vi "Configure Trigger (CAN).vi"(0 "VISA resource name":refnum<visa-resource-name>, 1 "Identifier":T2={"ID Mode (0: Standard)"=0, "ID Value (XXXXXXXXXXX)"="XXXXXXXXXXX"} {"ID Mode (0: Standard)" items=["Standard", "Extended"]}, 2 "Data":T1={"Data Size (1)"=1, "Data Value (XXXXXXXX)"="XXXXXXXX"}, 5 "Trigger Source (9: Bus 1)":u16(ring)=9 items=["Bus 1"=9, "Bus 2"=10, "Bus 3"=11, "Bus 4"=12], 7 "Condition (0: Start of Frame)":u16(ring) items=["Start of Frame", "Type of Frame", "Identifier", "Data", "ID & Data", "End of Frame", "Missing Ack"], 9 "Frame Type (0: Data)":u16(ring) items=["Data", "Remote", "Error", "Overload"], 11 "error in (no error)":errorcluster) -> (4 "VISA resource name out":refnum<visa-resource-name>, 15 "error out":errorcluster)   [LabVIEW 2013, in "Tektronix DPO MSO 2000 4000 Series.lvlib"]
doc: "Configures CAN trigger settings for an oscilloscope."
uses:
  Tektronix DPO MSO 2000 4000 Series.lvlib
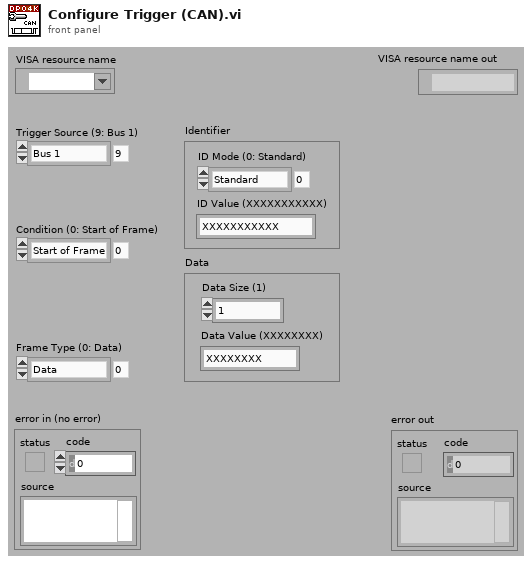
[diagram p1: front panel]
types:
  T1 = cluster{"Data Size (1)":i32, "Data Value (XXXXXXXX)":string}
  T2 = cluster{"ID Mode (0: Standard)":u16, "ID Value (XXXXXXXXXXX)":string}
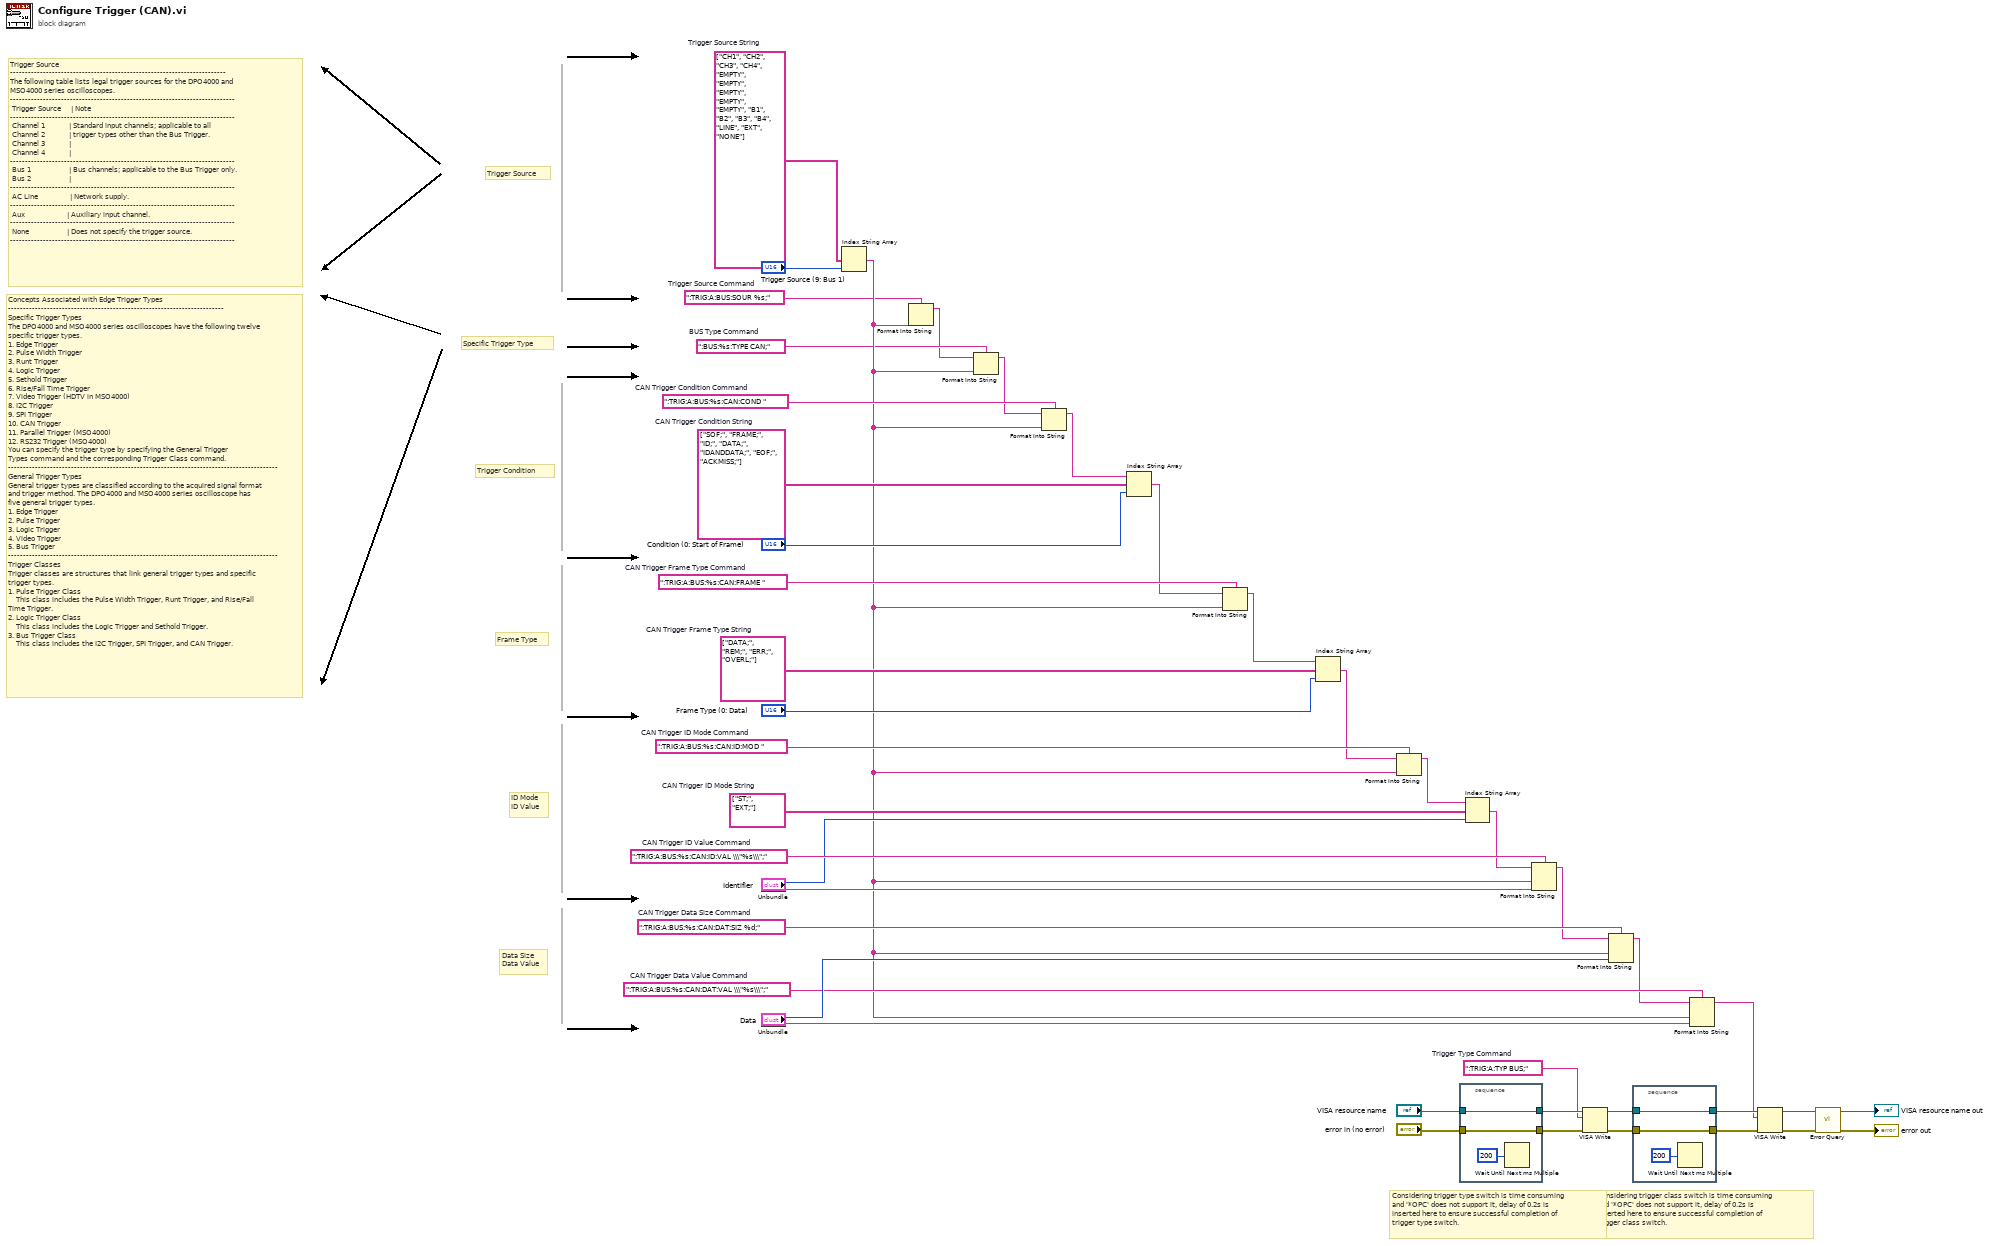
[diagram p0: block diagram]
diagram:
  w11 = string[] ["CH1", "CH2", "CH3", "CH4", "EMPTY", "EMPTY", "EMPTY", "EMPTY", "EMPTY", "B1", "B2", "B3", "B4", "LINE", "EXT", "NONE"]  # Trigger Source String
  w10 = ":TRIG:A:BUS:SOUR %s;"  # Trigger Source Command
  w20 = ":TRIG:A:TYP BUS;"  # Trigger Type Command
  w24 = ":TRIG:A:BUS:%s:CAN:DAT:VAL \\\"%s\\\";"  # CAN Trigger Data Value Command
  w29 = ":TRIG:A:BUS:%s:CAN:DAT:SIZ %d;"  # CAN Trigger Data Size Command
  w32 = ":TRIG:A:BUS:%s:CAN:ID:VAL \\\"%s\\\";"  # CAN Trigger ID Value Command
  w34 = string[] ["ST;", "EXT;"]  # CAN Trigger ID Mode String
  w36 = ":TRIG:A:BUS:%s:CAN:ID:MOD "  # CAN Trigger ID Mode Command
  w39 = string[] ["DATA;", "REM;", "ERR;", "OVERL;"]  # CAN Trigger Frame Type String
  w41 = ":TRIG:A:BUS:%s:CAN:FRAME "  # CAN Trigger Frame Type Command
  w43 = string[] ["SOF;", "FRAME;", "ID;", "DATA;", "IDANDDATA;", "EOF;", "ACKMISS;"]  # CAN Trigger Condition String
  w45 = ":TRIG:A:BUS:%s:CAN:COND "  # CAN Trigger Condition Command
  w9 = ":BUS:%s:TYPE CAN;"  # BUS Type Command
  # "Concepts Associated with Edge Trigger Types\n------------------------------------------------------------------------\nSpecific Trigger Types\nThe DPO4000 and MSO4000 series oscilloscopes have the following twelve specific trigger types.\n1. Edge Trigger\n2. Pulse Width Trigger\n3. Runt Trigger\n4. Logic Trigger\n5. Sethold Trigger\n6. Rise/Fall Time Trigger\n7. Video Trigger (HDTV in MSO4000)\n8. I2C Trigger\n9. SPI Trigger\n10. CAN Trigger\n11. Parallel Trigger (MSO4000)\n12. RS232 Trigger (MSO4000)\nYou can specify the trigger type by specifying the General Trigger \nTypes command and the corresponding Trigger Class command.\n------------------------------------------------------------------------------------------\nGeneral Trigger Types \nGeneral trigger types are classified according to the acquired signal format and trigger method. The DPO4000 and MSO4000 series oscilloscope has five general trigger types.\n1. Edge Trigger\n2. Pulse Trigger\n3. Logic Trigger\n4. Video Trigger\n5. Bus Trigger\n------------------------------------------------------------------------------------------\nTrigger Classes\nTrigger classes are structures that link general trigger types and specific trigger types.\n1. Pulse Trigger Class\n    This class includes the Pulse Width Trigger, Runt Trigger, and Rise/Fall Time Trigger.\n2. Logic Trigger Class\n    This class includes the Logic Trigger and Sethold Trigger.\n3. Bus Trigger Class\n    This class includes the I2C Trigger, SPI Trigger, and CAN Trigger."
  # "Trigger Source\n------------------------------------------------------------------------\nThe following table lists legal trigger sources for the DPO4000 and MSO4000 series oscilloscopes.\n---------------------------------------------------------------------------\n Trigger Source     | Note                                                           \n---------------------------------------------------------------------------\n Channel 1            | Standard input channels; applicable to all      \n Channel 2            | trigger types other than the Bus Trigger.         \n Channel 3            |     \n Channel 4            |\n---------------------------------------------------------------------------\n Bus 1                   | Bus channels; applicable to the Bus Trigger only.\n Bus 2                   | \n---------------------------------------------------------------------------\n AC Line                | Network supply.\n---------------------------------------------------------------------------\n Aux                     | Auxiliary input channel.\n---------------------------------------------------------------------------\n None                   | Does not specify the trigger source.\n---------------------------------------------------------------------------"
  # "Data Size\nData Value"
  # "ID Mode\nID Value"
  # "Frame Type"
  # "Trigger Condition"
  # "Specific Trigger Type"
  # "Trigger Source"
  # "Considering trigger class switch is time consuming\nand '*OPC' does not support it, delay of 0.2s is \ninserted here to ensure successful completion of\ntrigger class switch."
  # "Considering trigger type switch is time consuming\nand '*OPC' does not support it, delay of 0.2s is \ninserted here to ensure successful completion of\ntrigger type switch."
  n1 = Unbundle("Identifier") -> ("ID Mode (0: Standard)"=w30:u16, "ID Value (XXXXXXXXXXX)"=w31:string)
  n2 = Unbundle("Data") -> ("Data Size (1)"=w25:i32, "Data Value (XXXXXXXX)"=w26:string)
  n3 = Index String Array(1:"Trigger Source (9: Bus 1)", 2:w11) -> (0:w12:string)  [unwired: 1 in]
  n4 = Format Into String(format string=w10, w12) -> (resulting string=w6:string)  [unwired: 2 in, 1 out]
  n5 = Format Into String(format string=w9, initial string=w6, w12) -> (resulting string=w8:string)  [unwired: 1 in, 1 out]
  n6 = Format Into String(format string=w45, initial string=w8, w12) -> (resulting string=w44:string)  [unwired: 1 in, 1 out]
  n7 = Index String Array(1:"Condition (0: Start of Frame)", 2:w43, 3:w44) -> (0:w7:string)
  n8 = Format Into String(format string=w41, initial string=w7, w12) -> (resulting string=w40:string)  [unwired: 1 in, 1 out]
  n9 = Index String Array(1:"Frame Type (0: Data)", 2:w39, 3:w40) -> (0:w35:string)
  n10 = Format Into String(format string=w36, initial string=w35, w12) -> (resulting string=w33:string)  [unwired: 1 in, 1 out]
  n11 = stacked-sequence {
    tunnel: "VISA resource name" -> [w48]
    tunnel: [w48] -> w22
    tunnel: "error in (no error)" -> [w47]
    tunnel: [w47] -> w21
    frame #0 {
      n12 = Wait Until Next ms Multiple(millisecond multiple=u32 200) -> ()  [unwired: 1 out]
    }
  }
  n13 = Index String Array(1:w30, 2:w34, 3:w33) -> (0:w13:string)
  n14 = Format Into String(format string=w32, initial string=w13, w12, w31) -> (resulting string=w28:string)  [unwired: 1 in, 1 out]
  n15 = VISA Write(VISA resource name=w22, write buffer=w20, error in (no error)=w21) -> (VISA resource name out=w19:refnum<visa-resource-name>, error out=w18:errorcluster)  [unwired: 1 out]
  n16 = Format Into String(format string=w29, initial string=w28, w12, w25) -> (resulting string=w23:string)  [unwired: 1 in, 1 out]
  n17 = stacked-sequence {
    tunnel: w19 -> [w51]
    tunnel: [w51] -> w14
    tunnel: w18 -> [w50]
    tunnel: [w50] -> w17
    frame #0 {
      n18 = Wait Until Next ms Multiple(millisecond multiple=u32 200) -> ()  [unwired: 1 out]
    }
  }
  n19 = Format Into String(format string=w24, initial string=w23, w12, w26) -> (resulting string=w5:string)  [unwired: 1 in, 1 out]
  n20 = VISA Write(VISA resource name=w14, write buffer=w5, error in (no error)=w17) -> (VISA resource name out=w16:refnum<visa-resource-name>, error out=w15:errorcluster)  [unwired: 1 out]
  n21 = call "Error Query.vi"("error in (no error)"=w15, "VISA resource name"=w16) -> ("error out"=→"error out":errorcluster, "VISA resource name out"=→"VISA resource name out":refnum<visa-resource-name>)  [unwired: 6 in, 2 out]
